vi "Head_OrientationBoundary.vi"(11 "Angle in":dbl) -> (3 "Angle out":dbl)   [LabVIEW 2017]
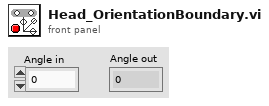
[diagram p1: front panel]
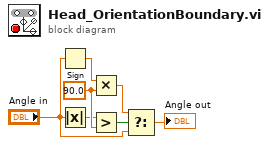
[diagram p0: block diagram]
diagram:
  w5 = 90.0 ("y")
  n1 = Sign(1:"Angle in") -> (0:w3:dbl)
  n2 = Absolute Value(x="Angle in") -> (abs(x)=w1:dbl)
  n3 = Multiply(x=w3, y=w5) -> (x*y=w4:dbl)
  n4 = Greater?(x=w1, y=w5) -> (0:w2:bool)
  n5 = Select(t=w4, s=w2, f="Angle in") -> (s? t:f=→"Angle out":dbl)
